vi "VI-FILE-F.S.D.S. MASTER.vi"() -> ()   [LabVIEW 2013]
panel:
  out "Drawing Room\nREMOTE triigger 4":bool
  out "Chamber\nFIRE detection 4":bool
  out "Chamber\nFIRE detection 3":bool
  out "Chamber\nFIRE detection 2":bool
  out "Drawing Room\nREMOTE triigger 3":bool
  out "REMOTE triigger 3":bool
  out "REMOTE triigger 3":bool
  out "Drawing Room\nREMOTE triigger 2":bool
  in  "Drawing Room\nLOCAL trigger":bool
  in  "Dining Room\nLOCAL trigger":bool
  in  "Library\nLOCAL trigger":bool
  in  "Chamber\nLOCAL trigger":bool
  in  "Drawing Room\nARMED switch":bool
  in  "Dining Room\nARMED switch":bool
  in  "Library\nARMED switch":bool
  in  "Chamber\nARMED switch":bool
  out "Chamber\nFIRE detection":bool
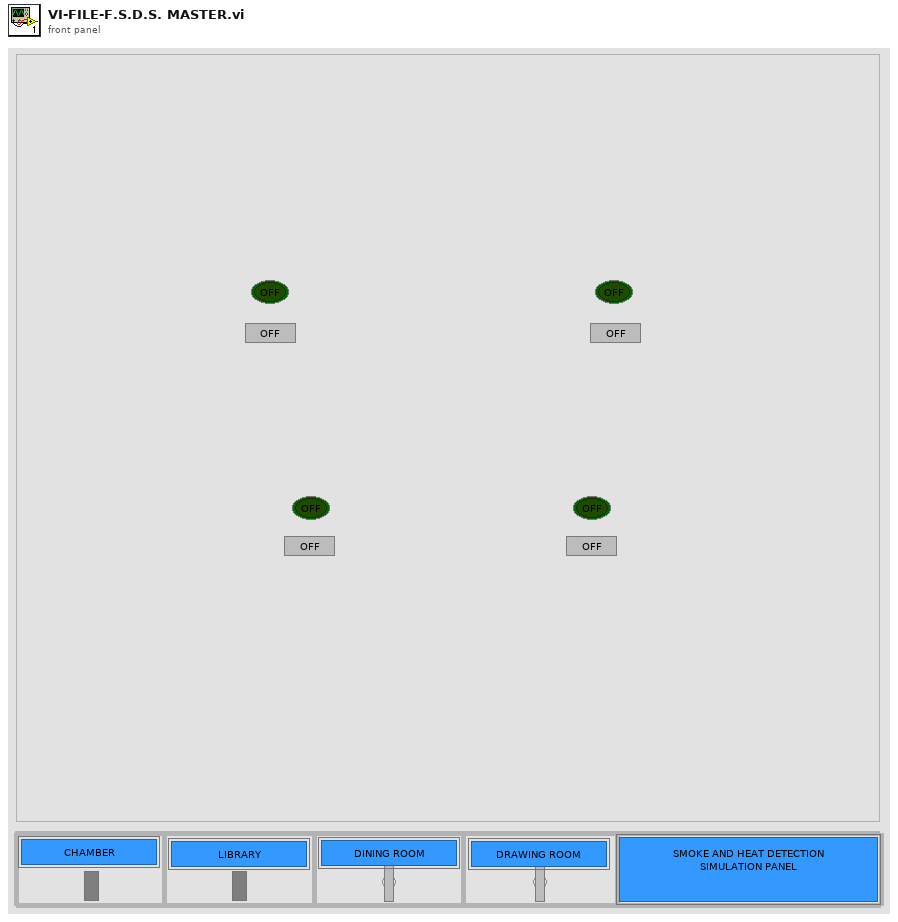
[diagram p1: front panel]
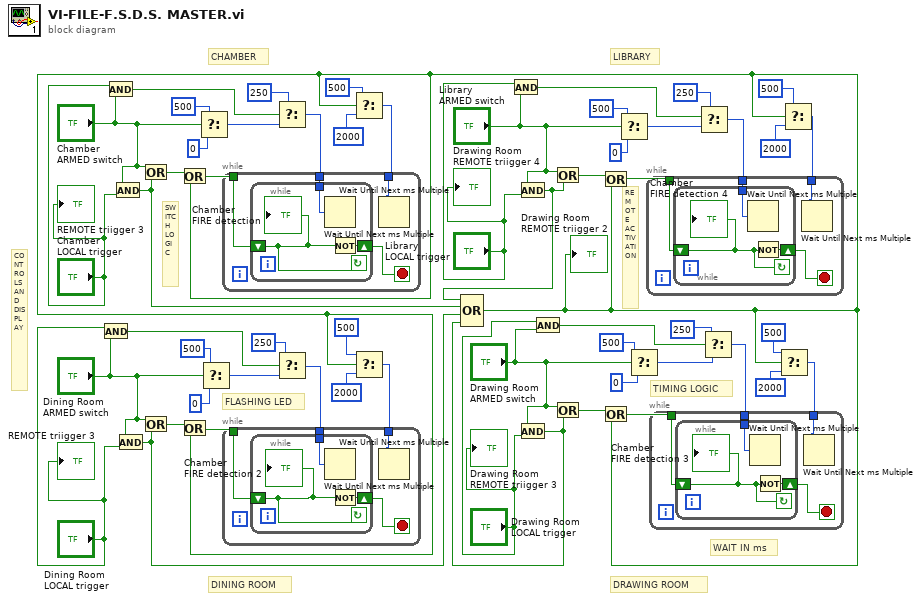
[diagram p0: block diagram]
diagram:
  # "WAIT IN ms"
  # "TIMING LOGIC"
  # "SWITCH LOGIC"
  # "CONTROLS AND DISPLAY"
  # "REMOTE ACTIVATION"
  # "FLASHING LED"
  # "DRAWING ROOM"
  # "DINING ROOM"
  # "LIBRARY"
  # "CHAMBER"
  n1 = And(x="Dining Room\nLOCAL trigger", y="Dining Room\nARMED switch") -> (x .and. y?=w8:bool)
  n2 = And(x="Chamber\nLOCAL trigger", y="Chamber\nARMED switch") -> (x .and. y?=w13:bool)
  n3 = And(x="Chamber\nARMED switch", y="Chamber\nLOCAL trigger") -> (x .and. y?=w57:bool)
  n4 = And(x="Dining Room\nARMED switch", y="Dining Room\nLOCAL trigger") -> (x .and. y?=w56:bool)
  n5 = Or(x="Chamber\nARMED switch", y=w57) -> (x .or. y?=w52:bool)
  n6 = Or(x="Dining Room\nARMED switch", y=w56) -> (x .or. y?=w51:bool)
  n7 = Select(t=u32 500, s="Chamber\nARMED switch", f=u32 0) -> (s? t:f=w43:u32)
  n8 = Select(t=u32 500 ("millisecond timer value"), s="Dining Room\nARMED switch", f=u32 0) -> (s? t:f=w29:u32)
  n9 = Select(t=u32 250, s=w13, f=w43) -> (s? t:f=w15:u32)
  n10 = Select(t=u32 250, s=w8, f=w29) -> (s? t:f=w31:u32)
  n11 = And(x="Library\nLOCAL trigger", y="Library\nARMED switch") -> (x .and. y?=w10:bool)
  n12 = And(x="Library\nARMED switch", y="Library\nLOCAL trigger") -> (x .and. y?=w16:bool)
  n13 = And(x="Drawing Room\nARMED switch", y="Drawing Room\nLOCAL trigger") -> (x .and. y?=w55:bool)
  n14 = Compound Arithmetic op=OR ("REMOTE trigger")(w16, w57, w56, w55) -> (w1:bool)
  "Drawing Room\nREMOTE triigger 2" <- w1
  n15 = Or(x=w52, y=w1) -> (x .or. y?=w50:bool)
  n16 = Or(x=w51, y=w1) -> (x .or. y?=w47:bool)
  n17 = Select(t=u32 500, s=w1, f=u32 2000 ("millisecond timer value")) -> (s? t:f=w17:u32)
  n18 = while {
    tunnel: w50 -> [w60]
    tunnel: w17 -> [w59]
    tunnel: w15 -> [w58]
    stop <- w61 stop-if-true
    n19 = while {
      shift-right: [w64] -> w61
      shift-left: w60 -> [w63]
      tunnel: w58 -> [w62]
      stop <- w63 continue-if-true
      n20 = Wait Until Next ms Multiple(millisecond multiple=w62) -> ()  [unwired: 1 out]
      n21 = Not(x=w63) -> (.not. x?=w64:bool)
      "Chamber\nFIRE detection" <- w63
    }
    n22 = Wait Until Next ms Multiple(millisecond multiple=w59) -> ()  [unwired: 1 out]
  }
  n23 = Select(t=u32 500, s=w1, f=u32 2000 ("millisecond timer value")) -> (s? t:f=w33:u32)
  n24 = while {
    tunnel: w47 -> [w67]
    tunnel: w33 -> [w66]
    tunnel: w31 -> [w65]
    stop <- w68 stop-if-true
    n25 = while {
      shift-right: [w71] -> w68
      shift-left: w67 -> [w69]
      tunnel: w65 -> [w70]
      stop <- w69 continue-if-true
      n26 = Wait Until Next ms Multiple(millisecond multiple=w70) -> ()  [unwired: 1 out]
      n27 = Not(x=w69) -> (.not. x?=w71:bool)
      "Chamber\nFIRE detection 2" <- w69
    }
    n28 = Wait Until Next ms Multiple(millisecond multiple=w66) -> ()  [unwired: 1 out]
  }
  n29 = And(x="Drawing Room\nLOCAL trigger", y="Drawing Room\nARMED switch") -> (x .and. y?=w7:bool)
  n30 = Or(x="Library\nARMED switch", y=w16) -> (x .or. y?=w54:bool)
  n31 = Or(x="Drawing Room\nARMED switch", y=w55) -> (x .or. y?=w53:bool)
  n32 = Or(x=w54, y=w1) -> (x .or. y?=w49:bool)
  n33 = Or(x=w53, y=w1) -> (x .or. y?=w48:bool)
  n34 = Select(t=u32 500, s="Library\nARMED switch", f=u32 0) -> (s? t:f=w37:u32)
  n35 = Select(t=u32 500, s="Drawing Room\nARMED switch", f=u32 0) -> (s? t:f=w24:u32)
  n36 = Select(t=u32 250 ("millisecond timer value"), s=w10, f=w37) -> (s? t:f=w36:u32)
  n37 = Select(t=u32 250, s=w7, f=w24) -> (s? t:f=w20:u32)
  n38 = Select(t=u32 500, s=w1, f=u32 2000 ("millisecond timer value")) -> (s? t:f=w19:u32)
  n39 = while {
    tunnel: w48 -> [w74]
    tunnel: w19 -> [w73]
    tunnel: w20 -> [w72]
    stop <- w75 stop-if-true
    n40 = while {
      shift-right: [w78] -> w75
      shift-left: w74 -> [w76]
      tunnel: w72 -> [w77]
      stop <- w76 continue-if-true
      n41 = Wait Until Next ms Multiple(millisecond multiple=w77) -> ()  [unwired: 1 out]
      n42 = Not(x=w76) -> (.not. x?=w78:bool)
      "Chamber\nFIRE detection 3" <- w76
    }
    n43 = Wait Until Next ms Multiple(millisecond multiple=w73) -> ()  [unwired: 1 out]
  }
  n44 = Select(t=u32 500, s=w1, f=u32 2000 ("millisecond timer value")) -> (s? t:f=w18:u32)
  n45 = while {
    tunnel: w49 -> [w81]
    tunnel: w18 -> [w80]
    tunnel: w36 -> [w79]
    stop <- w82 stop-if-true
    n46 = while {
      shift-right: [w85] -> w82
      shift-left: w81 -> [w83]
      tunnel: w79 -> [w84]
      stop <- w83 continue-if-true
      n47 = Wait Until Next ms Multiple(millisecond multiple=w84) -> ()  [unwired: 1 out]
      n48 = Not(x=w83) -> (.not. x?=w85:bool)
      "Chamber\nFIRE detection 4" <- w83
    }
    n49 = Wait Until Next ms Multiple(millisecond multiple=w80) -> ()  [unwired: 1 out]
  }
  "REMOTE triigger 3" <- "Dining Room\nLOCAL trigger"
  "Drawing Room\nREMOTE triigger 3" <- "Drawing Room\nLOCAL trigger"
  "REMOTE triigger 3" <- "Chamber\nLOCAL trigger"
  "Drawing Room\nREMOTE triigger 4" <- "Library\nLOCAL trigger"
